vi "Find Ajdacent Pulses.vi"(11 "Array in":bool[](array[boolean])) -> (3 "Array out":bool[](array[boolean]))   [LabVIEW 2023]
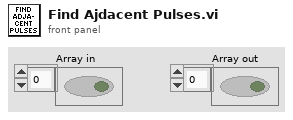
[diagram p1: front panel]
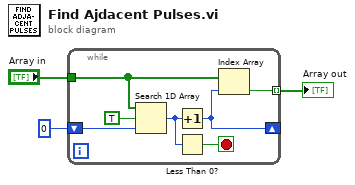
[diagram p0: block diagram]
diagram:
  n1 = while {
    tunnel: "Array in" -> [w8]
    shift-right: [w4] -> _
    shift-left: 0 ("start index (0)") -> [w10]
    tunnel: [w7] -> w2 mode=indexing
    stop <- w9 stop-if-true
    n2 = Search 1D Array(1D array=w8, element=TRUE, start index (0)=w10) -> (index of element=w6:i32)
    n3 = Increment(x=w6) -> (x+1=w4:i32)
    n4 = Less Than 0?(x=w6) -> (x < 0?=w9:bool)
    n5 = Index Array(array=w8, index=w4) -> (element=w7:bool)
  }
  "Array out" <- w2
